vi "Configure Clock Recovery (First Order PLL.vi"(7 "Enable Clock Recovery (T: Enable)":bool=TRUE, 8 "error in (no error)":errorcluster, 9 "Loop Bandwidth (1.5E+6 Hz)":dbl=1500000.0, 10 "Data Rate (2.5E+9 bits/s)":dbl=2500000000.0, 11 "VISA resource name":refnum<visa-resource-name>) -> (0 "error out":errorcluster, 3 "VISA resource name out":refnum<visa-resource-name>)   [LabVIEW 2015, in "Agilent 2000 3000 X-Series.lvlib"]
doc: "Configures the clock recovery using the DSP-modeled response of an\nideal first-order hardware PLL.\n\n<b>Note:</b>\nThis VI is specific to the 6000-X Series oscilloscopes. These features are not available on other models. Use <b>Configure Math Function Characteristics</b> and <b>Configure Math Function Source</b> before running this vi to set <b>Clock Recovery</b> as the math function and select the desired source."
uses:
  Agilent 2000 3000 X-Series.lvlib
panel:
  # "Note:\nThis VI has been obsoleted from the driver  and is included for \ncompatibility with existing applications.  New applications should use the\nConfigure Clock Recovery (First Order PLL) VI."
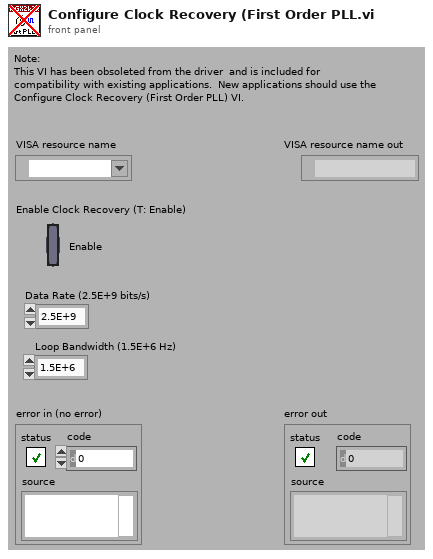
[diagram p1: front panel]
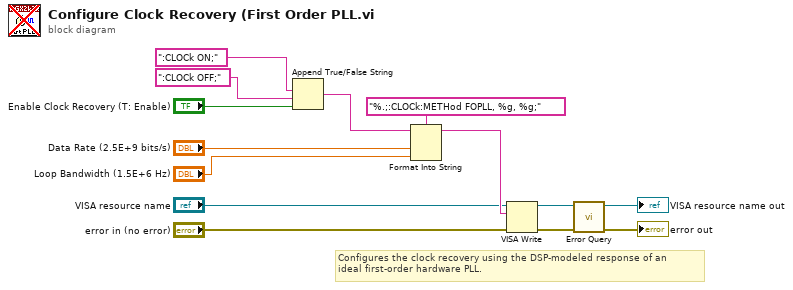
[diagram p0: block diagram]
diagram:
  # "Configures the clock recovery using the DSP-modeled response of an\nideal first-order hardware PLL."
  n1 = Append True/False String(1:"Enable Clock Recovery (T: Enable)", 2:":CLOCk OFF;", 3:":CLOCk ON;") -> (0:w11:string)  [unwired: 1 in]
  n2 = Format Into String(format string="%.;:CLOCk:METHod FOPLL, %g, %g;", initial string=w11, "Data Rate (2.5E+9 bits/s)", "Loop Bandwidth (1.5E+6 Hz)") -> (resulting string=w10:string)  [unwired: 1 in, 1 out]
  n3 = VISA Write(VISA resource name="VISA resource name", write buffer=w10, error in (no error)="error in (no error)") -> (VISA resource name out=w4:refnum<visa-resource-name>, error out=w3:errorcluster)  [unwired: 1 out]
  n4 = call "Error Query.vi"("error in (no error)"=w3, "VISA resource name"=w4) -> ("error out"=→"error out":errorcluster, "VISA resource name out"=→"VISA resource name out":refnum<visa-resource-name>)  [unwired: 6 in, 2 out]
